vi "Initialize Front Panel.vi"(8 "error in (no error)":errorcluster, 11 "Test Executive Builder Dirty Dot View in":refnum<class "Test Executive Builder Dirty Dot View.lvclass">) -> (0 "error out":errorcluster, 3 "Test Executive Builder Dirty Dot View out":refnum<class "Test Executive Builder Dirty Dot View.lvclass">)   [LabVIEW 2017, in "Test Executive Builder Dirty Dot View.lvclass"]
doc: "<License>\nCopyright © 2017 Composed Systems, LLC | All rights reserved\nwww.composed.io\n\nAuthor: Ethan Stern <ethan.stern@composed.io>\n\nThis software is provided \"AS IS\" WITHOUT WARRANTIES, either express or implied, AND IS FOR EDUCATIONAL PURPOSES ONLY.\n</License>"
uses:
  Test Executive Builder Dirty Dot View.lvclass
  <vilib>/gpm_packages/@cs/mva-viewable/Source/IViewable/IViewable/IViewable.lvclass
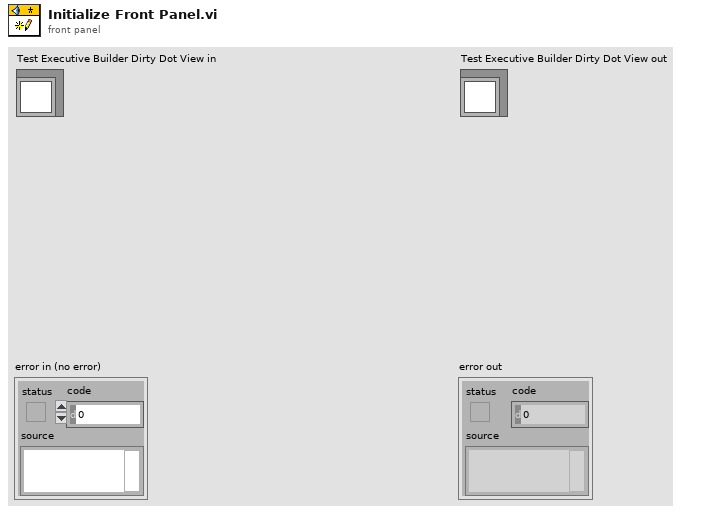
[diagram p1: front panel]
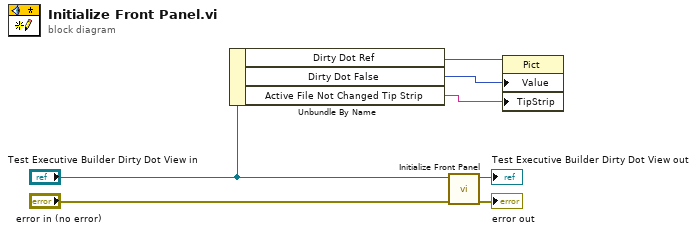
[diagram p0: block diagram]
diagram:
  n1 = Unbundle By Name("Test Executive Builder Dirty Dot View in") -> ("Dirty Dot Ref"=w3:refnum<vi>, "Dirty Dot False"=w2:picture, "Active File Not Changed Tip Strip"=w1:string)
  n2 = call-parent "Initialize Front Panel.vi"("error in (no error)"="error in (no error)", "IViewable in"="Test Executive Builder Dirty Dot View in") -> ("error out"=→"error out":errorcluster, "IViewable out"=→"Test Executive Builder Dirty Dot View out":refnum<class "Test Executive Builder Dirty Dot View.lvclass">)  [unwired: 8 in]
  n3 = property class="Pict"(reference=w3, "Value"=w2, "TipStrip"=w1) -> ()  [unwired: 1 in, 2 out]
